vi "Tree for configuration.vi"() -> ()   [LabVIEW 2023]
uses:
  e76aca29-4a87-4efb-9029-2c4417c4dd51.vi
  <vilib>/Utility/Data Type/NI_Data Type.lvlib
panel:
  out "Static Out":T1
  in  "MCL":T1
  in  "CL1":T2
  in  "CL2":T3={"s8"="erty", "i2"=77, "i9"=33, "b2"=TRUE, "b3"=FALSE}
  in  "Read(f) Write(t)":bool
  in  "Team Files Folder":path
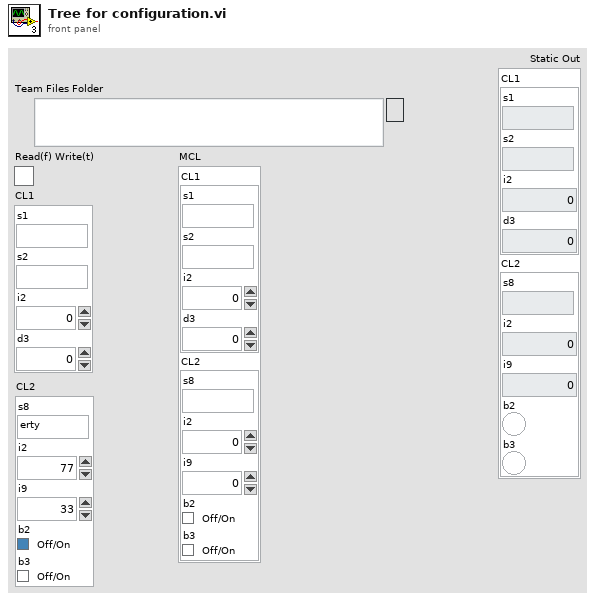
[diagram p1: front panel]
types:
  T1 = cluster{"CL1":cluster{"s1":string, "s2":string, "i2":i32, "d3":dbl}, "CL2":cluster{"s8":string, "i2":i32, "i9":i32, "b2":bool, "b3":bool}}
  T2 = cluster{"s1":string, "s2":string, "i2":i32, "d3":dbl}
  T3 = cluster{"s8":string, "i2":i32, "i9":i32, "b2":bool, "b3":bool}
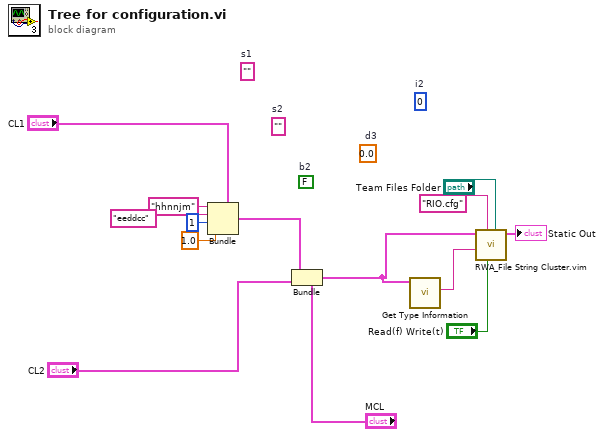
[diagram p0: block diagram]
diagram:
  (unwired) FALSE  # b2
  (unwired) 0.0  # d3
  (unwired) 0  # i2
  (unwired) ""  # s2
  (unwired) ""  # s1
  n1 = Bundle(cluster="CL1", "s1"="hhnnjm", "s2"="eeddcc" ("s1"), "i2"=1, "d3"=1.0) -> (w9:T2)
  n2 = Bundle(cluster="MCL", "CL1"=w9, "CL2"="CL2") -> (w3:T1)
  n3 = call <vilib>:"Get Type Information.vi"("variant"=w3) -> ("name"=w2:string)  [unwired: 6 in, 4 out]
  n4 = call "RWA_File String Cluster.vim"("Message Out"="Team Files Folder", "Read(f) Write(t)"="Read(f) Write(t)", 7:"RIO.cfg" ("File Name"), "Section Name"=w2, "Config"=w3) -> ("Config Out"=→"Static Out":T1)  [unwired: 3 in, 3 out]
